vi "WriteStartFreq.vi"(8 "error in (no error)":errorcluster, 11 "ChirpEIS in":refnum<class "ChirpEIS.lvclass">) -> (0 "error out":errorcluster, 3 "ChirpEIS out":refnum<class "ChirpEIS.lvclass">)   [LabVIEW 2014, in "ChirpEIS.lvclass"]
uses:
  ChirpEIS.lvclass
  ChirpEIS.lvclass/ChirpEIS.ctl
  States.ctl
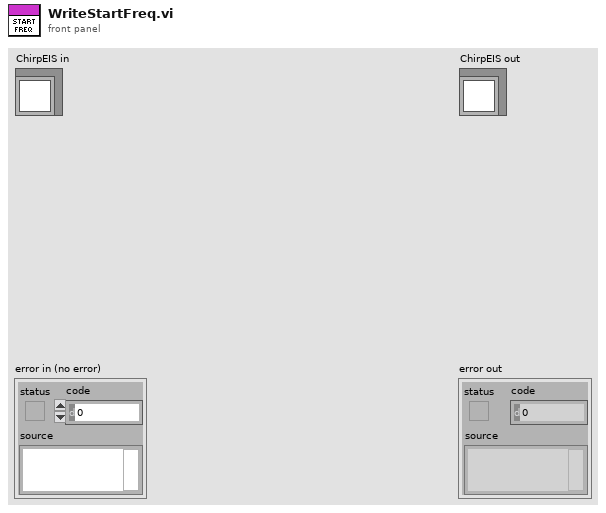
[diagram p1: front panel]
types:
  T1 = typedef "States.ctl" = enum16{"AddDuration", "AddFreq", "CreateNewFile", "Wait", "IncreaseVoltage", "DFT", "ChirpMeasurement", "Initialize", "Ternimate"}
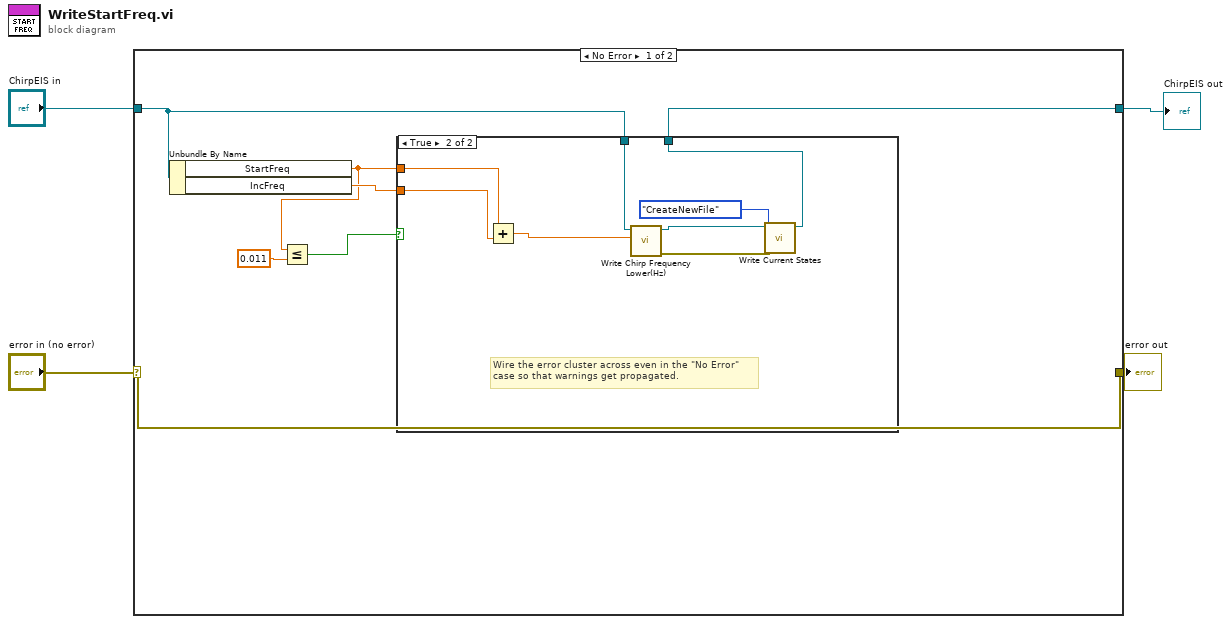
[diagram p0: block diagram]
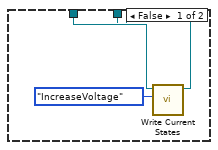
[diagram p2: hidden frame]
diagram:
  n1 = case shown="No Error" "error in (no error)" {
    selector: "error in (no error)" -> [w11 w24]
    tunnel: [w11 w24] -> w3
    tunnel: [w7 w23] -> w1
    tunnel: "ChirpEIS in" -> [w8 w23]
    frame No Error {
      n2 = Unbundle By Name(w8) -> ("StartFreq"=w5:dbl, "IncFreq"=w6:dbl)
      n3 = Less Or Equal?(x=w5, y=0.011) -> (x <= y?=w9:bool)
      n4 = case shown="True" w9 {
        tunnel: w8 -> [w14 w22]
        tunnel: [w12 w16] -> w7
        tunnel: w6 -> [_ w21]
        tunnel: w5 -> [_ w20]
        frame False {
          n5 = call-dynamic "Write Current States.vi"("Enum"=States."IncreaseVoltage", "ChirpEIS in"=w14) -> ("ChirpEIS out"=w12:refnum<class "ChirpEIS.lvclass">)  [unwired: 7 in, 2 out]
        }
        frame True {
          # "Wire the error cluster across even in the \"No Error\"\ncase so that warnings get propagated."
          n6 = Add(x=w20, y=w21) -> (x+y=w19:dbl)
          n7 = call-dynamic "Write Chirp Frequency Lower(Hz).vi"("Chirp Frequency Lower(Hz)"=w19, "ChirpEIS in"=w22) -> ("error out"=w17:errorcluster, "ChirpEIS out"=w18:refnum<class "ChirpEIS.lvclass">)  [unwired: 8 in]
          n8 = call-dynamic "Write Current States.vi"("error in (no error)"=w17, "Enum"=States."CreateNewFile", "ChirpEIS in"=w18) -> ("ChirpEIS out"=w16:refnum<class "ChirpEIS.lvclass">)  [unwired: 6 in, 2 out]
        }
      }
    }
    frame Error {
    }
  }
  "error out" <- w3
  "ChirpEIS out" <- w1
